vi "event_connecting.vi"(11 "message":string) -> ()   [LabVIEW 2014]
uses:
  QwaveSys_ESP8266/QwaveSys_ESP8266.lvlib
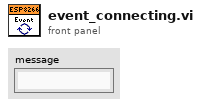
[diagram p1: front panel]
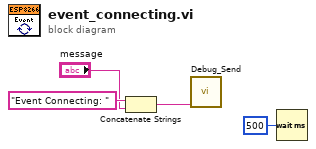
[diagram p0: block diagram]
diagram:
  n1 = Concatenate Strings("Event Connecting: " ("string"), "message") -> (w2:string)
  n2 = call "Debug_Send.vi"("DATA"=w2) -> ()  [unwired: 11 in]
  n3 = Wait (ms)(milliseconds to wait=u32 500) -> ()  [unwired: 1 out]
